vi "gas_manifold_control.vi"() -> ()   [LabVIEW 2014]
uses:
  <vilib>/Instr/_visa.llb/VISA Configure Serial Port (Instr).vi
  <vilib>/FieldPoint/Polymorphic Write.llb/FP Write (Boolean).vi
panel:
  out "read_error":bool
  in  "allow_multiple_valves":bool=TRUE
  in  "valve0":bool
  in  "valve1":bool
  in  "valve2":bool
  in  "valve3":bool
  in  "valve4":bool
  in  "valve5":bool
  out "valve_state":bool[](array[boolean])=[TRUE, FALSE, FALSE, FALSE, FALSE, FALSE]
  in  "STOP AND SAVE STATE":bool
  out "manifold pressure [torr]":dbl(knob) scale=0.0..1023.0
  out "number":dbl format="%#_6f"
  in  "read_pressure?":bool=TRUE
  # "0: vac\n1: N2\n2: He\n3: Ar\n4: SF6\n5: Xe/Kr"
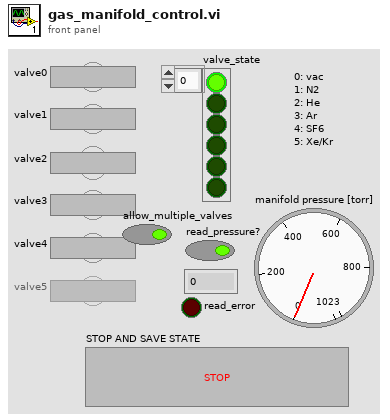
[diagram p1: front panel]
types:
  T1 = enum16{"open", "replace", "create", "open or create", "replace or create", "replace or create with confirmation"}
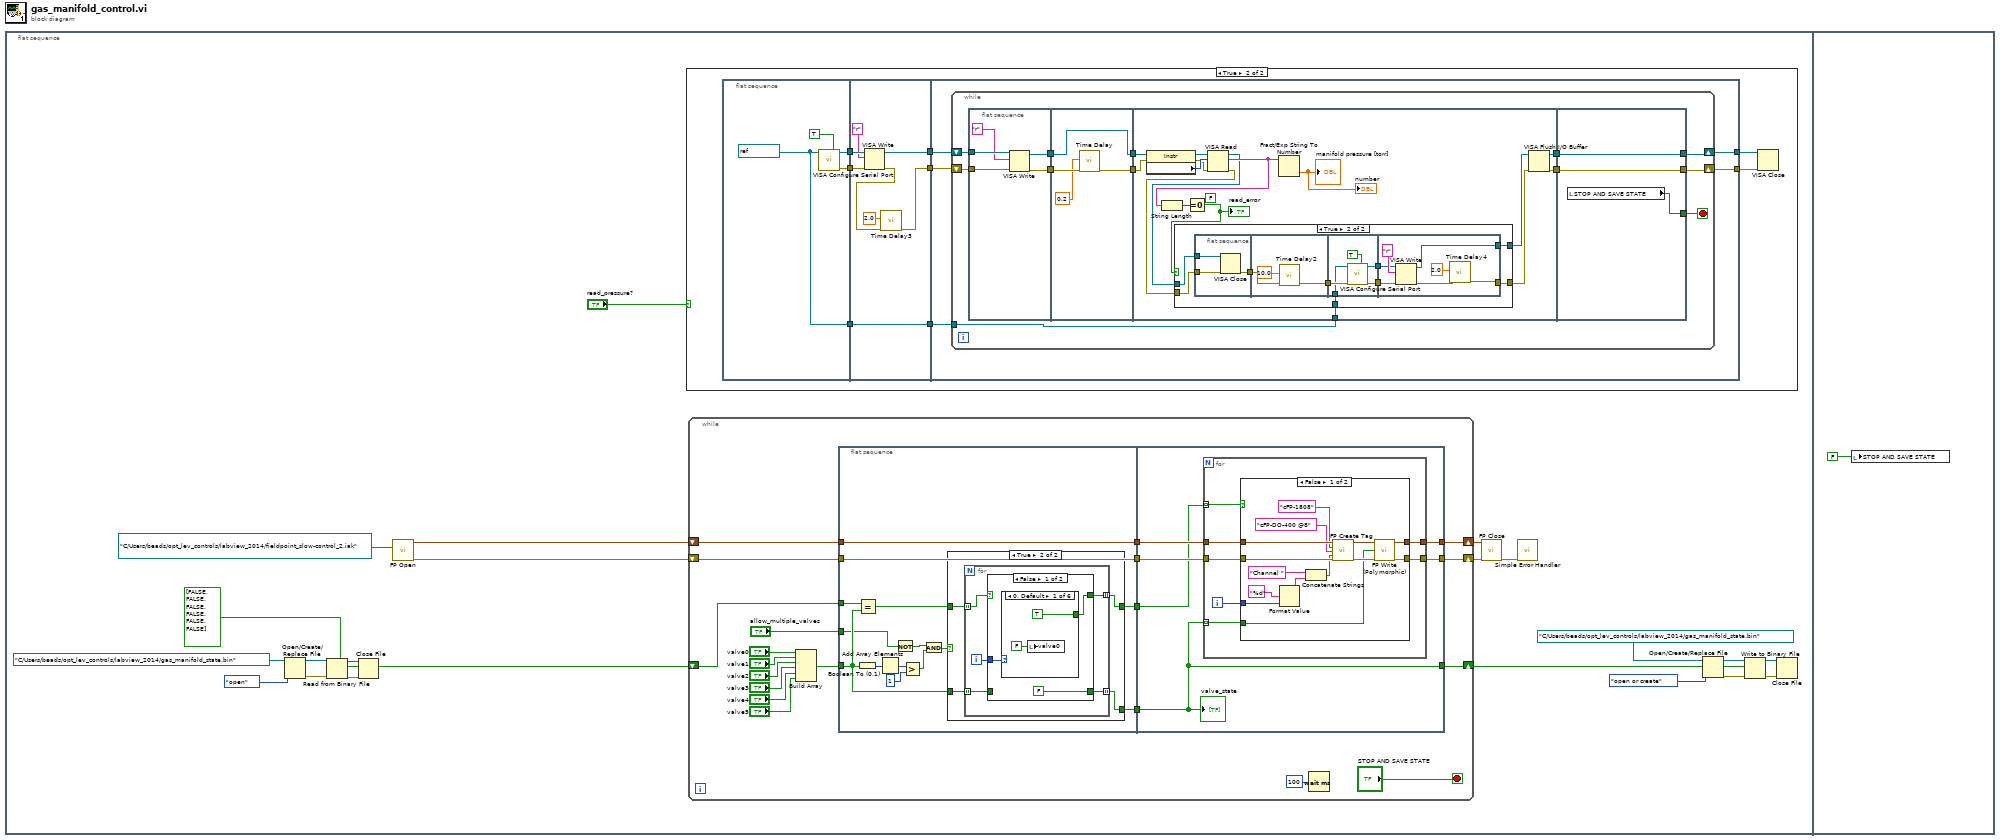
[diagram p0: block diagram]
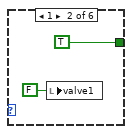
[diagram p3: hidden frame]
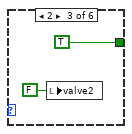
[diagram p4: hidden frame]
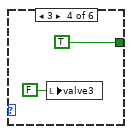
[diagram p5: hidden frame]
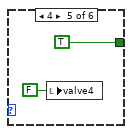
[diagram p6: hidden frame]
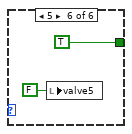
[diagram p7: hidden frame]
diagram:
  n1 = flat-sequence {
    frame #0 {
      n2 = Open/Create/Replace File(file path (use dialog)=path "C:/Users/beads/opt_lev_controls/labview_2014/gas_manifold_state.bin", operation (0:open)=T1."open") -> (refnum out=w7:refnum<file>, error out=w8:errorcluster)  [unwired: 4 in, 1 out]
      n3 = Read from Binary File(5:bool[] [FALSE, FALSE, FALSE, FALSE, FALSE, FALSE], 8:w8, 11:w7) -> (0:w6:errorcluster, 2:w2:bool[], 3:w5:refnum<file>)  [unwired: 3 in, 1 out]
      n4 = Close File(refnum=w5, error in=w6) -> ()  [unwired: 2 out]
      n5 = call <vilib>:"FP Open.vi"("iak file path"=path "C:/Users/beads/opt_lev_controls/labview_2014/fieldpoint_slow-control_2.iak") -> ("FP refnum out"=w20:cluster{"server refnum":u32, "tag refnum":u32}, "error out"=w19:errorcluster)  [unwired: 13 in]
      n6 = case shown="True" "read_pressure?" {
        frame False {
        }
        frame True {
          n7 = flat-sequence {
            tunnel: [w124] -> w121
            tunnel: [w123] -> w119
            tunnel: [w122] -> w117
            tunnel: w121 -> [w130]
            tunnel: [w127] -> w120
            tunnel: w119 -> [w129]
            tunnel: [w131] -> w118
            tunnel: w117 -> [w133]
            tunnel: [w133] -> w116
            tunnel: w120 -> [w138]
            tunnel: w118 -> [w137]
            tunnel: w116 -> [w136]
            tunnel: [w135] -> w115
            tunnel: [w134] -> w114
            frame #0 {
              w122 = refnum<visa-resource-name> "COM8" ("VISA resource name")
              n8 = call-poly "VISA Configure Serial Port"("VISA resource name"=w122, "Enable Termination\nChar (T)"=TRUE ("Enable Termination\nChar (T)")) -> ("VISA resource name out"=w124:refnum<visa-resource-name>, "error out"=w123:errorcluster)  [unwired: 12 in]
            }
            frame #1 {
              n9 = VISA Write(VISA resource name=w130, write buffer="r", error in (no error)=w129) -> (VISA resource name out=w127:refnum<visa-resource-name>, error out=w128:errorcluster)  [unwired: 1 out]
              n10 = call "Time Delay3"("error in (no error)"=w128, "Delay Time (s)"=2.0) -> ("error out"=w131:errorcluster)  [unwired: 9 in]
            }
            frame #2 {
              n11 = while {
                shift-right: [w144] -> w135
                shift-left: w138 -> [w146]
                shift-right: [w143] -> w134
                shift-left: w137 -> [w145]
                tunnel: w136 -> [w139]
                stop <- w140 stop-if-true
                n12 = flat-sequence {
                  tunnel: [w155] -> w150
                  tunnel: [w154] -> w149
                  tunnel: w146 -> [w153]
                  tunnel: w145 -> [w152]
                  tunnel: w150 -> [w159]
                  tunnel: [w158] -> w148
                  tunnel: w149 -> [w158]
                  tunnel: [w157] -> w147
                  tunnel: w148 -> [w175]
                  tunnel: w147 -> [w171]
                  tunnel: [w170] -> w142
                  tunnel: [w169] -> w141
                  tunnel: w139 -> [w163]
                  tunnel: [w206] -> w143
                  tunnel: [w207] -> w144
                  tunnel: w142 -> [w207]
                  tunnel: w141 -> [w206]
                  tunnel: [w205] -> w140
                  frame #0 {
                    n13 = VISA Write(VISA resource name=w153, write buffer="r", error in (no error)=w152) -> (VISA resource name out=w154:refnum<visa-resource-name>, error out=w155:errorcluster)  [unwired: 1 out]
                  }
                  frame #1 {
                    n14 = call "Time Delay"("error in (no error)"=w159, "Delay Time (s)"=0.2) -> ("error out"=w157:errorcluster)  [unwired: 9 in]
                  }
                  frame #2 {
                    (unwired) FALSE
                    n15 = property class="Instr"(reference=w175, error in=w171) -> (reference out=w174:refnum<visa-resource-name>, error out=w172:errorcluster, "Serial Settings:Number of Bytes at Serial Port"=w173:u32)
                    n16 = VISA Read(VISA resource name=w174, byte count=w173, error in (no error)=w172) -> (VISA resource name out=w164:refnum<visa-resource-name>, read buffer=w167:string, error out=w165:errorcluster)  [unwired: 1 out]
                    n17 = String Length(string=w167) -> (length=w166:i32)
                    n18 = Equal To 0?(x=w166) -> (x = 0?=w160:bool)
                    "read_error" <- w160
                    n19 = case shown="True" w160 {
                      tunnel: w165 -> [w176 w185]
                      tunnel: w164 -> [w177 w186]
                      tunnel: w163 -> [_ w182]
                      tunnel: [w177 w181] -> w162
                      tunnel: [w176 w180] -> w161
                      frame False {
                      }
                      frame True {
                        n20 = flat-sequence {
                          tunnel: w186 -> [w189]
                          tunnel: w185 -> [w188]
                          tunnel: [w187] -> w184
                          tunnel: w184 -> [w192]
                          tunnel: [w190] -> w183
                          tunnel: w183 -> [w197]
                          tunnel: w182 -> [w196]
                          tunnel: [w194] -> w179
                          tunnel: [w193] -> w178
                          tunnel: [w204] -> w180
                          tunnel: [w198] -> w181
                          tunnel: w179 -> [w202]
                          tunnel: w178 -> [w199]
                          frame #0 {
                            n21 = VISA Close(VISA resource name=w189, error in (no error)=w188) -> (error out=w187:errorcluster)
                          }
                          frame #1 {
                            n22 = call "Time Delay2"("error in (no error)"=w192, "Delay Time (s)"=10.0) -> ("error out"=w190:errorcluster)  [unwired: 9 in]
                          }
                          frame #2 {
                            n23 = call-poly "VISA Configure Serial Port"("VISA resource name"=w196, "Enable Termination\nChar (T)"=TRUE ("Enable Termination\nChar (T)"), "error in (no error)"=w197) -> ("VISA resource name out"=w193:refnum<visa-resource-name>, "error out"=w194:errorcluster)  [unwired: 11 in]
                          }
                          frame #3 {
                            n24 = VISA Write(VISA resource name=w199, write buffer="r", error in (no error)=w202) -> (VISA resource name out=w198:refnum<visa-resource-name>, error out=w200:errorcluster)  [unwired: 1 out]
                            n25 = call "Time Delay4"("error in (no error)"=w200, "Delay Time (s)"=2.0) -> ("error out"=w204:errorcluster)  [unwired: 9 in]
                          }
                        }
                      }
                    }
                    n26 = Fract/Exp String To Number(string=w167) -> (number=→"manifold pressure [torr]" →"number":dbl)  [unwired: 3 in, 1 out]
                    n27 = VISA Flush I/O Buffer(VISA resource name=w162, error in (no error)=w161) -> (VISA resource name out=w170:refnum<visa-resource-name>, error out=w169:errorcluster)  [unwired: 1 in]
                  }
                  frame #3 {
                    n28 = local read "STOP AND SAVE STATE"() -> (w205:bool)
                  }
                }
              }
            }
          }
          n29 = VISA Close(VISA resource name=w115, error in (no error)=w114) -> ()  [unwired: 1 out]
        }
      }
      n30 = while {
        shift-right: [w34] -> w17
        shift-left: w20 -> [w32]
        shift-right: [w33] -> w16
        shift-left: w19 -> [w31]
        shift-right: [w26] -> w1
        shift-left: w2 -> [w35]
        stop <- "STOP AND SAVE STATE" stop-if-true
        n31 = Build Array("valve0", "valve1", "valve2", "valve3", "valve4", "valve5") -> (w29:bool[])
        n32 = flat-sequence {
          tunnel: w29 -> [w51]
          tunnel: w31 -> [w55]
          tunnel: w32 -> [w56]
          tunnel: w35 -> [w54]
          tunnel: [w56] -> w28
          tunnel: [w55] -> w27
          tunnel: [w52] -> w25
          tunnel: "allow_multiple_valves" -> [w46]
          tunnel: [w47] -> w23
          tunnel: [w90] -> w34
          tunnel: [w89] -> w33
          tunnel: w28 -> [w88]
          tunnel: w27 -> [w87]
          tunnel: [w85] -> w26
          tunnel: w25 -> [w86]
          tunnel: w23 -> [w85]
          frame #0 {
            n33 = Boolean To (0,1)(Boolean=w51) -> (0, 1=w50:i16[])
            n34 = Equal?(x=w54, y=w51) -> (x = y?=w53:bool[])
            n35 = Add Array Elements(numeric array=w50) -> (sum=w49:i16)
            n36 = Not(x=w46) -> (.not. x?=w43:bool)
            n37 = Greater?(x=w49, y=i16 1) -> (0:w44:bool)
            n38 = And(x=w43, y=w44) -> (x .and. y?=w45:bool)
            n39 = case shown="True" w45 {
              tunnel: w53 -> [w58 w62]
              tunnel: [w58 w59] -> w52
              tunnel: w51 -> [w57 w61]
              tunnel: [w57 w60] -> w47
              frame False {
              }
              frame True {
                n40 = for {
                  tunnel: w62 -> [w67] mode=indexing
                  tunnel: w61 -> [w66] mode=indexing
                  tunnel: [w65] -> w60 mode=indexing
                  tunnel: [w64] -> w59 mode=indexing
                  i -> [w63]
                  n41 = case shown="False" w67 {
                    selector: w67 -> [_ w83]
                    tunnel: w66 -> [_ w84]
                    tunnel: [FALSE w84] -> w65
                    tunnel: [w69 w83] -> w64
                    tunnel: w63 -> [w70 _]
                    frame False {
                      n42 = case shown="0, Default" w70 {
                        tunnel: [TRUE TRUE TRUE TRUE TRUE TRUE] -> w69
                        frame 0, Default {
                          n43 = local write "valve0"(FALSE ("valve0")) -> ()
                        }
                        frame 1 {
                          n44 = local write "valve1"(FALSE ("valve0")) -> ()
                        }
                        frame 2 {
                          n45 = local write "valve2"(FALSE ("valve0")) -> ()
                        }
                        frame 3 {
                          n46 = local write "valve3"(FALSE ("valve0")) -> ()
                        }
                        frame 4 {
                          n47 = local write "valve4"(FALSE ("valve0")) -> ()
                        }
                        frame 5 {
                          n48 = local write "valve5"(FALSE ("valve0")) -> ()
                        }
                      }
                    }
                    frame True {
                    }
                  }
                }
              }
            }
          }
          frame #1 {
            n49 = for {
              tunnel: w86 -> [w97] mode=indexing
              tunnel: [w95] -> w90
              tunnel: [w94] -> w89
              tunnel: w88 -> [w93]
              tunnel: w87 -> [w92]
              tunnel: w85 -> [w91] mode=indexing
              i -> [w96]
              n50 = case shown="False" w97 {
                tunnel: w93 -> [w111 w113]
                tunnel: w92 -> [w110 w112]
                tunnel: [w105 w113] -> w95
                tunnel: [w104 w112] -> w94
                tunnel: w96 -> [w102 _]
                tunnel: w91 -> [w98 _]
                frame False {
                  n51 = Format Value(format string="%d", value (0)=w102) -> (output string=w100:string)  [unwired: 1 in]
                  n52 = Concatenate Strings("Channel " ("Item Name"), w100) -> (w99:string)
                  n53 = call <vilib>:"FP Create Tag.vi"("FP refnum in"=w111, "comm resource name"="cFP-1808" ("Comm Resource Name"), "device name"="cFP-DO-400 @8" ("Device Name"), "item name"=w99, "error in (no error)"=w110) -> ("FP refnum out"=w107:cluster{"server refnum":u32, "tag refnum":u32}, "error out"=w106:errorcluster)  [unwired: 9 in]
                  n54 = call-poly <vilib>:"FP Write (Polymorphic).vi"("FP refnum in"=w107, "value"=w98, "error in (no error)"=w106) -> ("FP refnum out"=w105:cluster{"server refnum":u32, "tag refnum":u32}, "error out"=w104:errorcluster)  [unwired: 10 in, 1 out]
                }
                frame True {
                }
              }
            }
            "valve_state" <- w85
          }
        }
        n55 = Wait (ms)(milliseconds to wait=u32 100) -> ()  [unwired: 1 out]
      }
      n56 = call <vilib>:"FP Close.vi"("FP refnum in"=w17, "error in (no error)"=w16) -> ("error out"=w18:errorcluster)  [unwired: 13 in]
      n57 = call <vilib>:"Simple Error Handler.vi"("error in (no error)"=w18) -> ()  [unwired: 4 in, 5 out]
      n58 = Open/Create/Replace File(file path (use dialog)=path "C:/Users/beads/opt_lev_controls/labview_2014/gas_manifold_state.bin", operation (0:open)=T1."open or create") -> (refnum out=w12:refnum<file>, error out=w13:errorcluster)  [unwired: 4 in, 1 out]
      n59 = Write to Binary File(file (use dialog)=w12, data=w1, error in=w13) -> (refnum out=w10:refnum<file>, error out=w11:errorcluster)  [unwired: 3 in, 1 out]
      n60 = Close File(refnum=w10, error in=w11) -> ()  [unwired: 2 out]
    }
    frame #1 {
      n61 = local write "STOP AND SAVE STATE"(FALSE ("STOP AND SAVE STATE")) -> ()
    }
  }
